vi "Read NET_HttpRequestMessage.vi"(8 "error in (no error)":errorcluster, 11 "HttpRequestMessage in":refnum<class "HttpRequestMessage.lvclass">) -> (0 "error out":errorcluster, 2 "NET_HttpRequestMessage":refnum<k24>, 3 "HttpRequestMessage out":refnum<class "HttpRequestMessage.lvclass">)   [LabVIEW 2018, in "HttpClient_NET.lvlib" / "HttpRequestMessage.lvclass"]
doc: "<b> </b> <b> </b>\nHttpClient_NET\nJustin Young - Viviota\nCopyright (c) 2021\nLicense: BSD"
uses:
  HttpRequestMessage.lvclass
  System.Net.Http
  HttpRequestMessage.lvclass/HttpRequestMessage.ctl
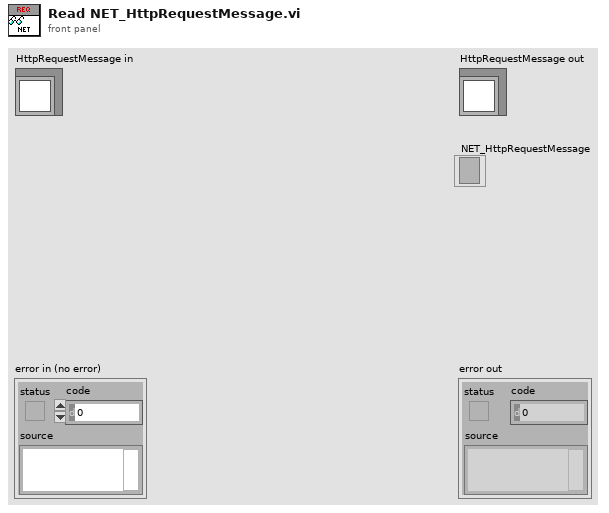
[diagram p1: front panel]
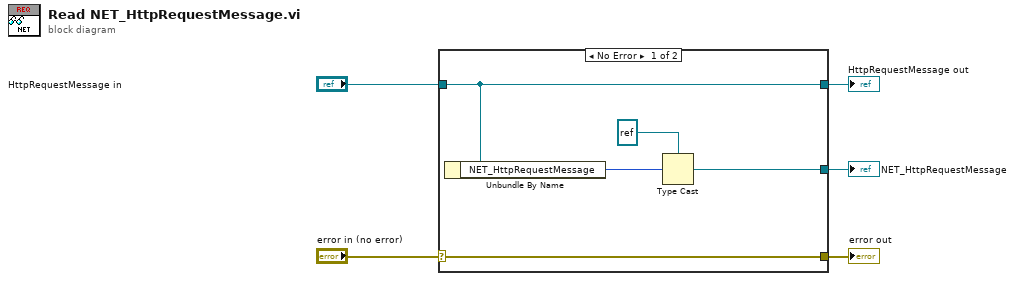
[diagram p0: block diagram]
diagram:
  n1 = case shown="No Error" "error in (no error)" {
    selector: "error in (no error)" -> [w10 w11]
    tunnel: [w10 w11] -> w4
    tunnel: [w9 w12] -> w2
    tunnel: "HttpRequestMessage in" -> [w9 w12]
    tunnel: [w7 _] -> w1
    frame No Error {
      n2 = Unbundle By Name(w9) -> ("NET_HttpRequestMessage"=w8:i64)
      n3 = Type Cast(type=refnum<k24> refnum ("NET_HttpRequestMessage"), x=w8) -> (*(type *) &x=w7:refnum<k24>)
    }
    frame Error {
    }
  }
  "error out" <- w4
  "HttpRequestMessage out" <- w2
  "NET_HttpRequestMessage" <- w1
